vi "channel operation tests.vi"() -> ()   [LabVIEW 2013, in "user code tests.lvlib"]
uses:
  user code tests.lvlib
  module/configuration/fixed channel tag bus module configuration.lvclass
panel:
  out "error out":errorcluster
  out "channels match":bool
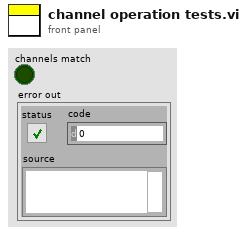
[diagram p1: front panel]
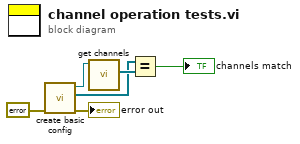
[diagram p0: block diagram]
diagram:
  n1 = call "create basic config.vi"("error in"=errorcluster {"status"=FALSE, "code"=0, "source"=""} ("error out")) -> ("error out"=→"error out":errorcluster, "generated channels"=w4:refnum<class "TBM channel.lvclass">[], "user tag bus module configuration out"=w3:refnum<class "fixed channel tag bus module configuration.lvclass">)  [unwired: 7 in, 1 out]
  n2 = call-dynamic "get channels.vi"("user tag bus module configuration In"=w3) -> ("channels"=w6:refnum<class "TBM channel.lvclass">[])  [unwired: 9 in, 1 out]
  n3 = Equal?(x=w4, y=w6) -> (x = y?=→"channels match":bool)
